vi "Inspection Program Write.vi"(8 "error in (no error)":errorcluster, 10 "IPF Folder":path, 11 "data in":T1) -> (0 "error out":errorcluster, 3 "data out":T1)   [LabVIEW 2013, in "Manipulate IPF.lvlib"]
uses:
  Manipulate IPF.lvlib
  3013/code/Modules/GUI/GUI_5/subPanels/edit/type_def/data.ctl
  3013/code/Modules/Configuration/type_def/Scan Params.ctl
  3013/code/Modules/Configuration/type_def/Profile Resolution.ctl
  3013/code/Modules/Preprocess Data/type_def/direction.ctl
  3013/code/Modules/Inspection/Data/Panel_class/type_def/Config File data.ctl
  3013/code/Modules/Inspection/type_def/Pos and Rot.ctl
  3013/code/Modules/Inspection/Data/PCB_class/type_def/PCB Params.ctl
  3013/code/Modules/Inspection/Data/Panel_class/type_def/BarCode Params.ctl
  3013/code/Modules/Barcode Reader/type_def/id.ctl
  3013/code/Modules/Inspection/Data/Panel_class/type_def/inspection data.ctl
  3013/code/Modules/Inspection/type_def/Range Limits.ctl
  <userlib>/_OpenG.lib/file/file.llb/Convert File Extension (String)__ogtk.vi
  3013/code/Modules/Configuration/Config.lvlib
  3013/code/Modules/Configuration/System/System.lvlib
  3013/code/Modules/Inspection/Data/Panel_class/Panel.lvclass
  3013/code/Modules/Inspection/Inspection.lvlib
  3013/code/Modules/Inspection/Data/PCB_class/PCB.lvclass
  3013/code/Modules/Barcode Reader/Barcode Reader.lvlib
  3013/code/Modules/GUI/GUI_5/subPanels/edit/edit.lvlib
  3013/code/Modules/Preprocess Data/PreProcess.lvlib
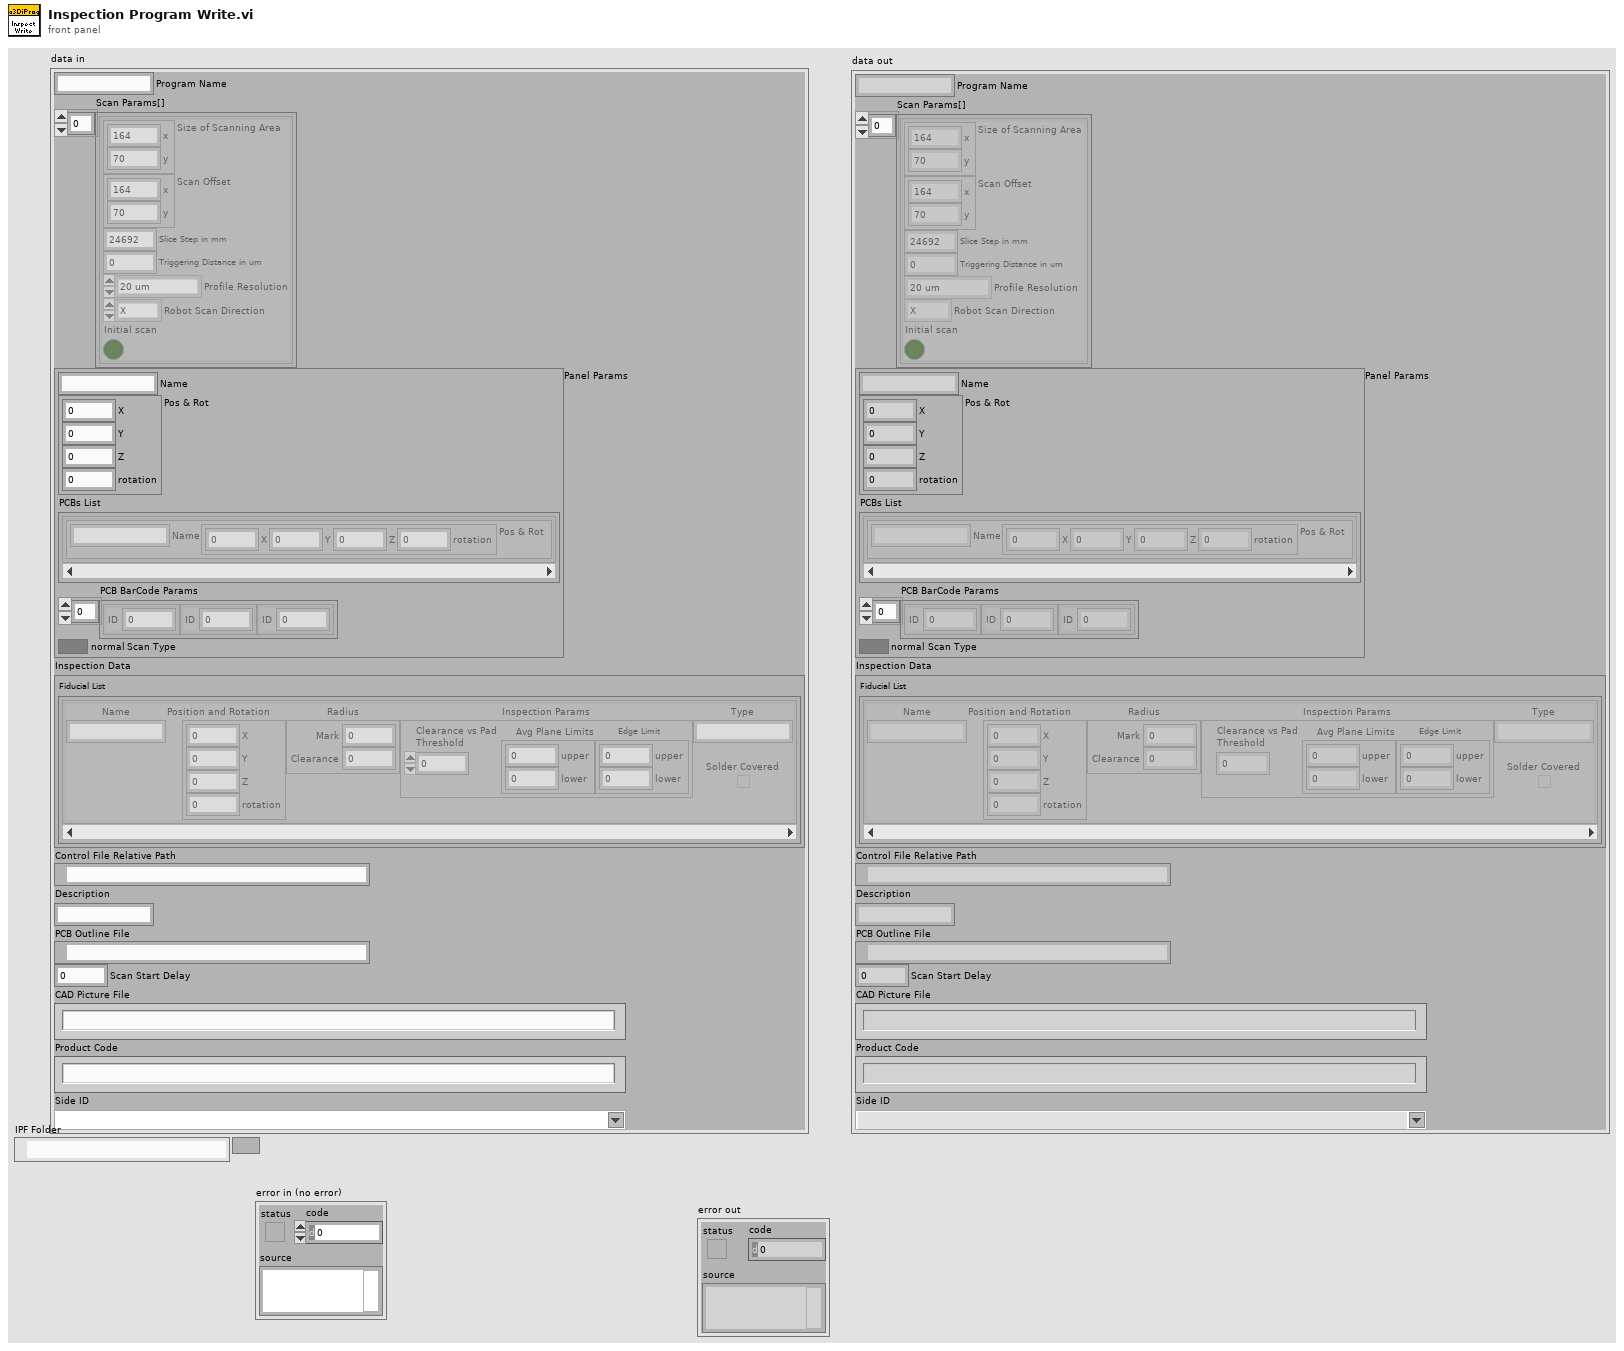
[diagram p1: front panel]
types:
  T1 = typedef "GUI.lvlib/subPanel.lvlib/edit.lvlib/data.ctl" = cluster{"Program Name":string, "Scan Params[]":T2[], "Panel Params":T5, "Inspection Data":T10, "Control File Relative Path":path, "Description":string, "PCB Outline File":path, "Scan Start Delay":dbl, "CAD Picture File":string, "Product Code":string, "Side ID":string}
  T2 = typedef "Config.lvlib/Scan Params.ctl" = cluster{"Size of Scanning Area":cluster{"x":dbl, "y":dbl}, "Scan Offset":cluster{"x":dbl, "y":dbl}, "Slice Step in mm":dbl, "Triggering Distance in mm":dbl, "Triggering Distance in um":dbl, "Profile Resolution":T3, "Version":string, "Robot Scan Direction":T4, "Initial scan":bool}
  T3 = typedef "Config.lvlib/Profile Resolution.ctl" = enum8{"20 um", "40 um"}
  T4 = typedef "PreProcess.lvlib/direction.ctl" = enum8{"X", "Y"}
  T5 = typedef "Inspection.lvlib/Panel.lvclass/Config File data.ctl" = cluster{"Name":string, "Pos & Rot":T6, "PCBs List":cluster{"PCB Params":T7}[], "PCB BarCode Params":T8[], "Scan Type":bool}
  T6 = typedef "Inspection.lvlib/Pos and Rot.ctl" = cluster{"X":dbl, "Y":dbl, "Z":dbl, "rotation":dbl}
  T7 = typedef "Inspection.lvlib/PCB.lvclass/PCB Params.ctl" = cluster{"Name":string, "Pos & Rot":T6}
  T8 = typedef "Inspection.lvlib/Panel.lvclass/BarCode Params.ctl" = cluster{"ID":T9}
  T9 = typedef "Barcode Reader.lvlib/id.ctl" = u8
  T10 = typedef "Inspection.lvlib/Panel.lvclass/inspection data.ctl" = cluster{"Fiducial List":cluster{"Name":string, "Position and Rotation":T6, "Radius":cluster{"Mark":dbl, "Clearance":dbl}, "Inspection Params":cluster{"Clearance vs Pad\nThreshold":dbl, "Avg Plane Limits":T11, "Edge Limit":T11}, "Type":string, "Solder Covered":bool}[]}
  T11 = typedef "Inspection.lvlib/Range Limits.ctl" = cluster{"upper":sgl, "lower":sgl}
  T12 = typedef "Config.lvlib/System.lvlib/config.ctl" = cluster{"a3Di station ID":string, "Customers ID":string, "User management file path":path, "Results Folder":path, "Scans Folder":path, "Product key (software protection)":string, "Logging Folder":path, "Robot Config":T13, "2D Scanner Config":T19, "2D Sensor Config":T20, "Inspection Config File":path, "Panel Config File":path, "a3Di Config File":path, "pw":string, "Inspection Prog File":path, "BCReaders Params":T29, "External Disks":T32, "Scanner Cal Tab":T34, "Scanner Cal Tab Flat":string, "Ticket Printing Config":T37, "calPCB CalTable":cluster{"Far":T39, "Near":T39}, "Side ID Alias":cluster{"Top":string, "Bottom":string}, "Calscan after":cluster{"Scans":T17, "Time (hours)":T18}}
  T13 = typedef "Config.lvlib/System.lvlib/Robot config.ctl" = cluster{"IP address":string, "Template Path Name":path, "Axes{}":T14, "Handler Position":T16, "Home robot after":cluster{"Scans":T17, "Time (hours)":T18}}
  T14 = typedef "Robot.lvlib/config.ctl" = T15[]
  T15 = typedef "Robot.lvlib/axis config.ctl" = cluster{"Name":string}
  T16 = typedef "Config.lvlib/System.lvlib/Handler Position.ctl" = cluster{"X_start":dbl, "Y_stop":dbl}
  T17 = typedef "Robot.lvlib/Last Homing max number of scans.ctl" = u32
  T18 = typedef "Robot.lvlib/Last homing max time.ctl" = dbl
  T19 = typedef "Config.lvlib/System.lvlib/2D Scanner.ctl" = cluster{"Calibration":string, "IP address":string}
  T20 = typedef "Config.lvlib/System.lvlib/2D Sensor config.ctl" = cluster{"multiScan":bool, "Sensor Cfg":T21, "Comm Interface":T24, "Ethernet Config":T25, "HighSpeed Port No":u16, "Start Req":T26, "Read Timeout(ms)":u32, "direction":T4, "Both Directions Scan":bool}
  T21 = typedef "Keyence LJ-V7000.lvlib/Sensors Config.ctl" = cluster{"X axis":cluster{"Reverse Direction":bool, "Pos Cal Params":T22}[], "Y axis":cluster{"Reverse Direction":bool, "Pos Cal Params":T22}[], "Rotation Offset":cluster{"x":dbl, "y":dbl, "z":dbl}}
  T22 = typedef "PreProcess.lvlib/Sensor Pos Calib Params.ctl" = cluster{"offset":cluster{"X":T23, "Y":T23, "Z":T23}, "angle":cluster{"XY":dbl, "XZ":dbl, "YZ":dbl}}
  T23 = typedef "Keyence LJ-V7000.lvlib/Sensor Units.ctl" = i32
  T24 = typedef "Keyence LJ-V7000.lvlib/Comm Interface.ctl" = enum8{"USB", "ETHERNET"}
  T25 = typedef "Keyence LJ-V7000.lvlib/Ethernet Config.ctl" = cluster{"IP Address":u8[], "Port No":u16}
  T26 = typedef "Keyence LJ-V7000.lvlib/High-Speed Comm Start Req.ctl" = cluster{"High-Speed Comm Start Pos":T27, "Read Profile Cnt":u32, "High-Speed Receive Ratio":T28}
  T27 = typedef "Keyence LJ-V7000.lvlib/High-Speed Comm Start Pos.ctl" = u8
  T28 = typedef "Keyence LJ-V7000.lvlib/High-Speed Receive Ratio.ctl" = u8
  T29 = typedef "Barcode Reader.lvlib/Multi Readers Config.ctl" = cluster{"Conveyor speed in mm/ms":dbl, "Distance between edge and sensor in mm":dbl, "BCReaders Params":T30[]}
  T30 = typedef "Barcode Reader.lvlib/msg data.ctl" = cluster{"ID":T9, "Enabled":bool, "IP Settings":T31}
  T31 = typedef "Barcode Reader.lvlib/IP settings.ctl" = cluster{"IP Address":string, "Port":u16}
  T32 = typedef "Mainenance.lvlib/external disk params.ctl" = cluster{"A":path, "B":path, "Active":T33, "Free Space Limit (%)":dbl}
  T33 = typedef "Mainenance.lvlib/disk_select.ctl" = enum16{"A", "B"}
  T34 = typedef "PreProcess.lvlib/Scanner Calibration Table.ctl" = cluster{"Robot X":cluster{"method":T35, "Cal Table":T36}, "Robot Y":cluster{"method":T35, "Sensors":cluster{"Cal Table":T36}[]}, "Orthogonality":dbl[]}
  T35 = typedef "calibration methode.ctl" = enum32{"nearest", "linear", "spline", "cubic Hermite", "Lagrange"}
  T36 = typedef "PreProcess.lvlib/Axis Calibration Table.ctl" = cluster{"in":dbl, "out":dbl}[]
  T37 = typedef "Results.lvlib/ticket printing config.ctl" = cluster{"Print Failed PCBs":bool, "Printer name (if empty then default)":string, "Max number of errors to print":i32, "Print Params":T38}
  T38 = typedef "Results.lvlib/print params.ctl" = cluster{"text options":cluster{"Italic":enum16{"Italic Unchanged", "Italic On", "Italic Off"}, "Strike Through":enum16{"Strike Through Unchanged", "Strike Through On", "Strike Through Off"}, "Underline":enum16{"Underline Unchanged", "Underline On", "Underline Off"}, "Bold":enum16{"Bold Unchanged", "Bold On", "Bold Off"}}, "font settings":cluster{"Charset":i16, "Weight":i16, "Name":string, "Size":string}, "Report Margins":cluster{"margins":cluster{"top":dbl, "left":dbl, "right":dbl, "bottom":dbl}, "measurement system":u16}, "Tab Width":cluster{"width":dbl, "measurement system":u16}}
  T39 = typedef "a3Di.lvlib/calPCB CalTable.ctl" = cluster{"method":T35, "calPCB CalTable [Sensor]":cluster{"Cal Table":T36}[]}
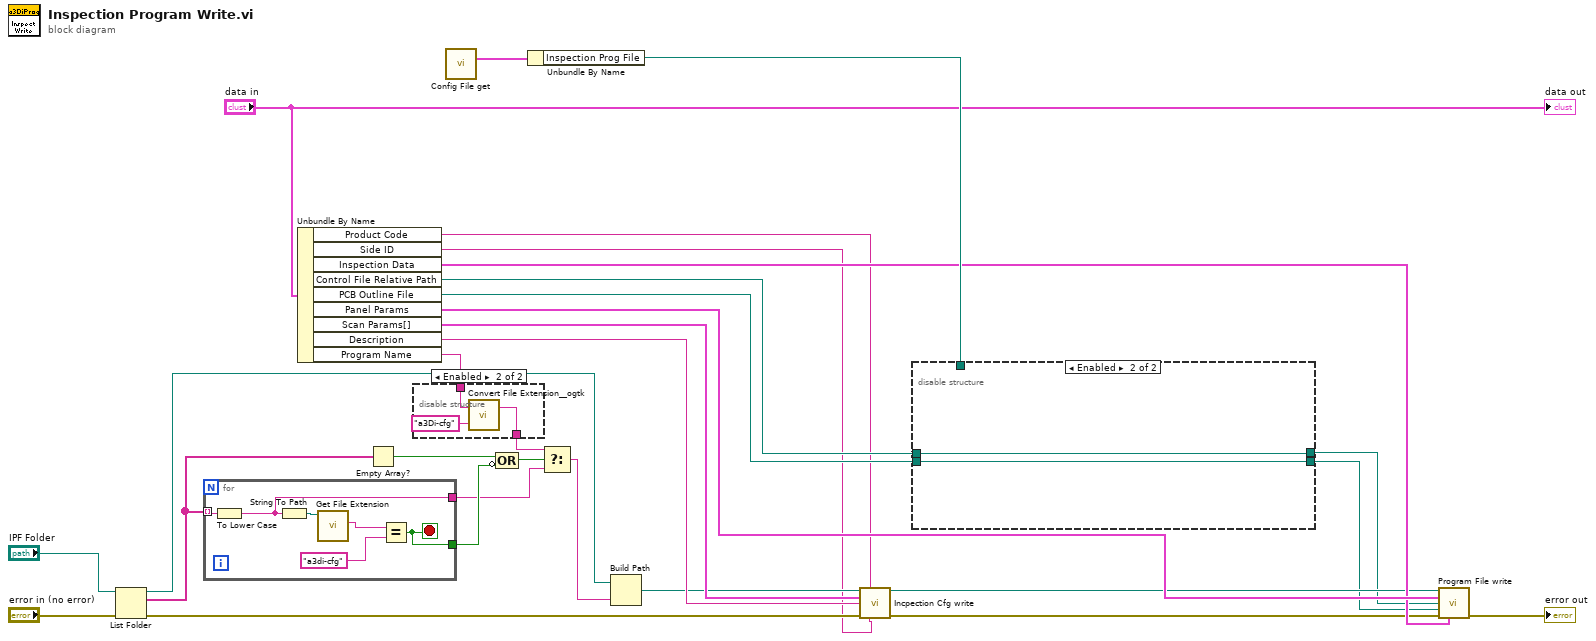
[diagram p0: block diagram]
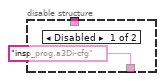
[diagram p2: hidden frame]
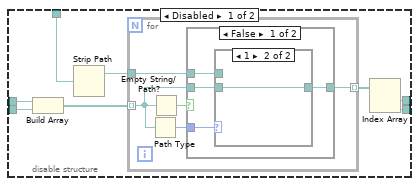
[diagram p3: hidden frame]
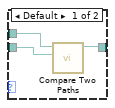
[diagram p4: hidden frame]
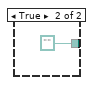
[diagram p5: hidden frame]
diagram:
  n1 = List Folder(path="IPF Folder", error in="error in (no error)") -> (path out=w21:path, filenames=w20:string[], error out=w23:errorcluster)  [unwired: 2 in, 1 out]
  n2 = for {
    tunnel: w20 -> [w30] mode=indexing
    tunnel: [w29] -> w16
    tunnel: [w31] -> w18
    stop <- w31 stop-if-true
    n3 = To Lower Case(string=w30) -> (all lower case string=w29:string)
    n4 = String To Path(string=w29) -> (path=w34:path)
    n5 = call <vilib>:"Get File Extension.vi"("file"=w34) -> ("lowercase file extension"=w33:string)  [unwired: 7 in, 3 out]
    n6 = Equal?(x=w33, y="a3di-cfg") -> (x = y?=w31:bool)
  }
  n7 = Unbundle By Name("data in") -> ("Product Code"=w2:string, "Side ID"=w1:string, "Inspection Data"=w8:T10, "Control File Relative Path"=w10:path, "PCB Outline File"=w9:path, "Panel Params"=w11:T5, "Scan Params[]"=w27:T2[], "Description"=w28:string, "Program Name"=w13:string)
  n8 = Empty Array?(array=w20) -> (empty?=w19:bool)
  n9 = disable-structure shown="Enabled" {
    disable-tunnel: w13 -> [_ w38]
    disable-tunnel: ["insp_prog.a3Di-cfg" ("name or relative path") w36] -> w12
    frame Disabled {
    }
    frame Enabled {
      n10 = call-poly <userlib>:"Convert File Extension__ogtk.vi"("new ending (none)"="a3Di-cfg", "file name"=w38) -> ("new filename"=w36:string)  [unwired: 1 out]
    }
  }
  n11 = call "Config File get.vi"() -> ("Configuration"=w25:T12)  [unwired: 14 in, 1 out]
  n12 = Compound Arithmetic op=OR(w19, invert w18) -> (w17:bool)
  n13 = Unbundle By Name(w25) -> ("Inspection Prog File"=w26:path)
  n14 = Select(t=w12, s=w17, f=w16) -> (s? t:f=w15:string)
  n15 = Build Path(base path=w21, name or relative path=w15) -> (appended path=w5:path)
  n16 = call "Incpection Cfg write.vi"("configuration file path"=w5, "Product Code"=w2, "Scan Params[]"=w27, "Description"=w28, "error in (no error)"=w23, "Side ID"=w1) -> ("error out"=w7:errorcluster)  [unwired: 9 in]
  n17 = disable-structure shown="Enabled" {
    disable-tunnel: w9 -> [w46 w61]
    disable-tunnel: w10 -> [w45 w62]
    disable-tunnel: [w41 w62] -> w4
    disable-tunnel: [w40 w61] -> w3
    disable-tunnel: w26 -> [w39 _]
    frame Disabled {
      n18 = Build Array(w45, w46) -> (w43:path[])
      n19 = Strip Path(path=w39) -> (stripped path=w44:path)  [unwired: 1 out]
      n20 = for {
        tunnel: w43 -> [w48] mode=indexing
        tunnel: [w50] -> w42 mode=indexing
        tunnel: w44 -> [w47]
        n21 = Path Type(1:w48) -> (0:w49:i16)
        n22 = Empty String/Path?(string/path=w48) -> (empty?=w51:bool)
        n23 = case shown="False" w51 {
          tunnel: [w53 path ""] -> w50
          tunnel: w49 -> [w55 _]
          tunnel: w48 -> [w54 _]
          tunnel: w47 -> [w52 _]
          frame False {
            n24 = case shown="1" w55 {
              tunnel: w54 -> [w57 w59]
              tunnel: [w58 w59] -> w53
              tunnel: w52 -> [w56 _]
              frame Default {
                n25 = call <vilib>:"Compare Two Paths.vi"("Path 2"=w57, "Path 1"=w56) -> ("Relative Path from 1 to 2"=w58:path)  [unwired: 6 in, 3 out]
              }
              frame 1 {
              }
            }
          }
          frame True {
          }
        }
      }
      n26 = Index Array(array=w42) -> (element #1=w41:path, element #2=w40:path)  [unwired: 2 in]
    }
    frame Enabled {
    }
  }
  n27 = call "Program File write.vi"("a3Di CFG file path"=w5, "Panel Params"=w11, "Control File Relative Path"=w4, "Outline File"=w3, "error in (no error)"=w7, "Inspection Data"=w8) -> ("error out"=→"error out":errorcluster)  [unwired: 9 in]
  "data out" <- "data in"
